vi "SiosIfmI2CRequestRead.vi"(1 "Amount of Bytes":i32, 2 "RAM Adress":i32, 3 "i2c Adress":i32, 4 "Device Number":i32) -> (0 "Success":i32)   [LabVIEW 2009]
uses:
  siosifm.dll
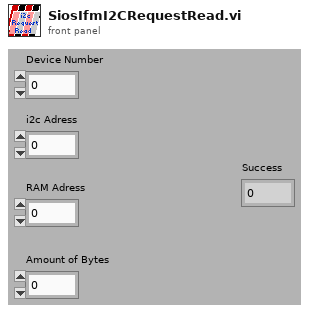
[diagram p1: front panel]
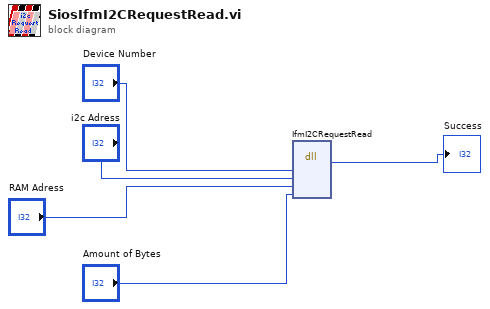
[diagram p0: block diagram]
diagram:
  n1 = dll-call lib="C:/WORK/Artem/RE-10/SIOS_IfmDLL/siosifm.dll" fn="IfmI2CRequestRead"("devNumber"="Device Number", "i2cAddr"="i2c Adress", "ramAddr"="RAM Adress", "count"="Amount of Bytes") -> ("success"=→"Success":i32)  [unwired: 7 in, 2 out]
